vi "Closest Point Delete.vi"(9 "Y in":dbl=359.5 format="%#_13g", 10 "X in":dbl=18.050867335505 format="%#_13g", 11 "All Lines":T1) -> (0 "min index(es)":i32, 1 "Y out":dbl, 2 "X out":dbl, 3 "output array":T1, 5 "Array size":i32)   [LabVIEW 2014]
uses:
  Libraries/Map Data Folder/All-Lines.ctl
  Libraries/Map Data Folder/LineCluster.ctl
  Libraries/Map Data Folder/LineConnection.ctl
  Libraries/Map Data Folder/Map Data.lvlib
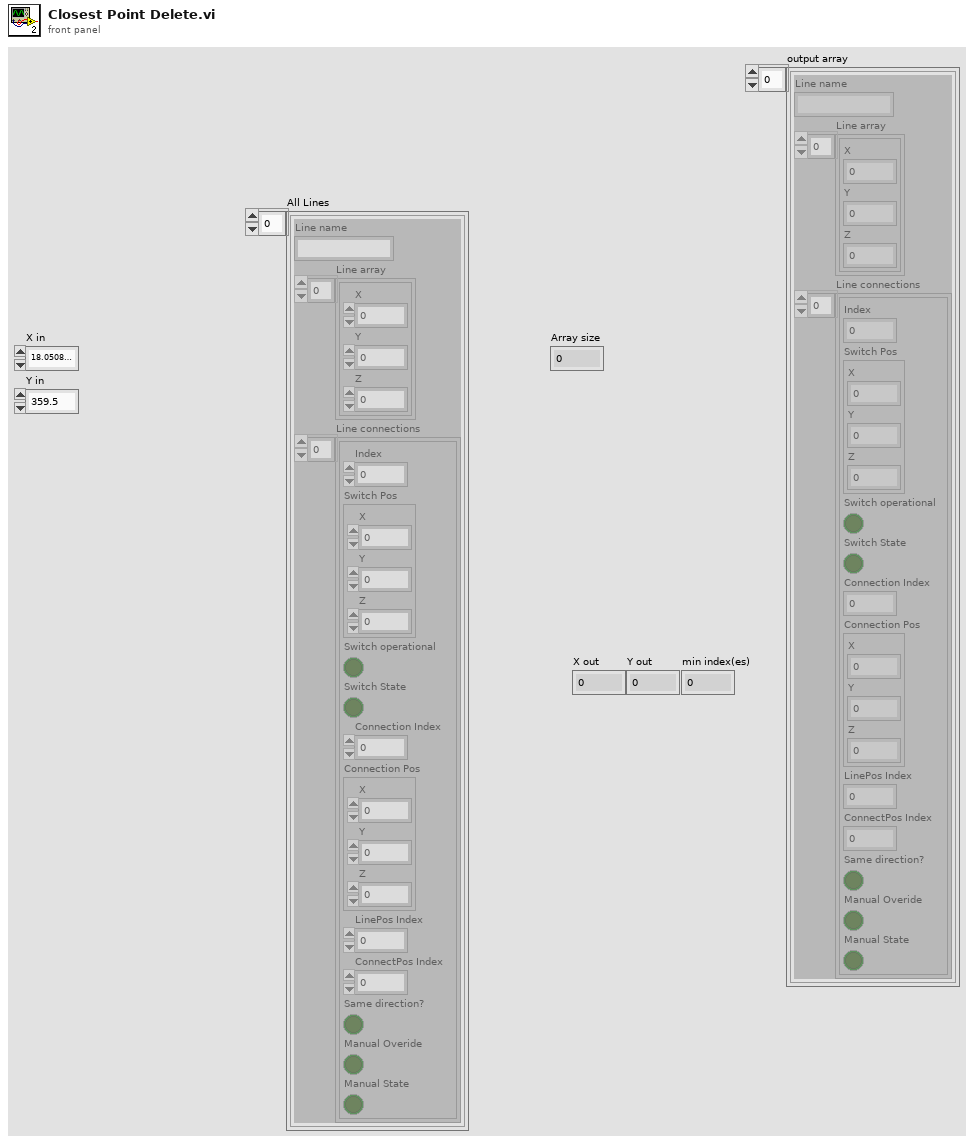
[diagram p1: front panel]
types:
  T1 = typedef "Map Data.lvlib/All-Lines.ctl" = T2[]
  T2 = typedef "Map Data.lvlib/LineCluster.ctl" = cluster{"Line name":string, "Line array":cluster{"X":dbl, "Y":dbl, "Z":dbl}[], "Line connections":T3[]}
  T3 = typedef "Map Data.lvlib/LineConnection.ctl" = cluster{"Index":i32, "Switch Pos":cluster{"X":dbl, "Y":dbl, "Z":dbl}, "Switch operational":bool, "Switch State":bool, "Connection Index":i32, "Connection Pos":cluster{"X":dbl, "Y":dbl, "Z":dbl}, "LinePos Index":i32, "ConnectPos Index":i32, "Same direction?":bool, "Manual Overide":bool, "Manual State":bool}
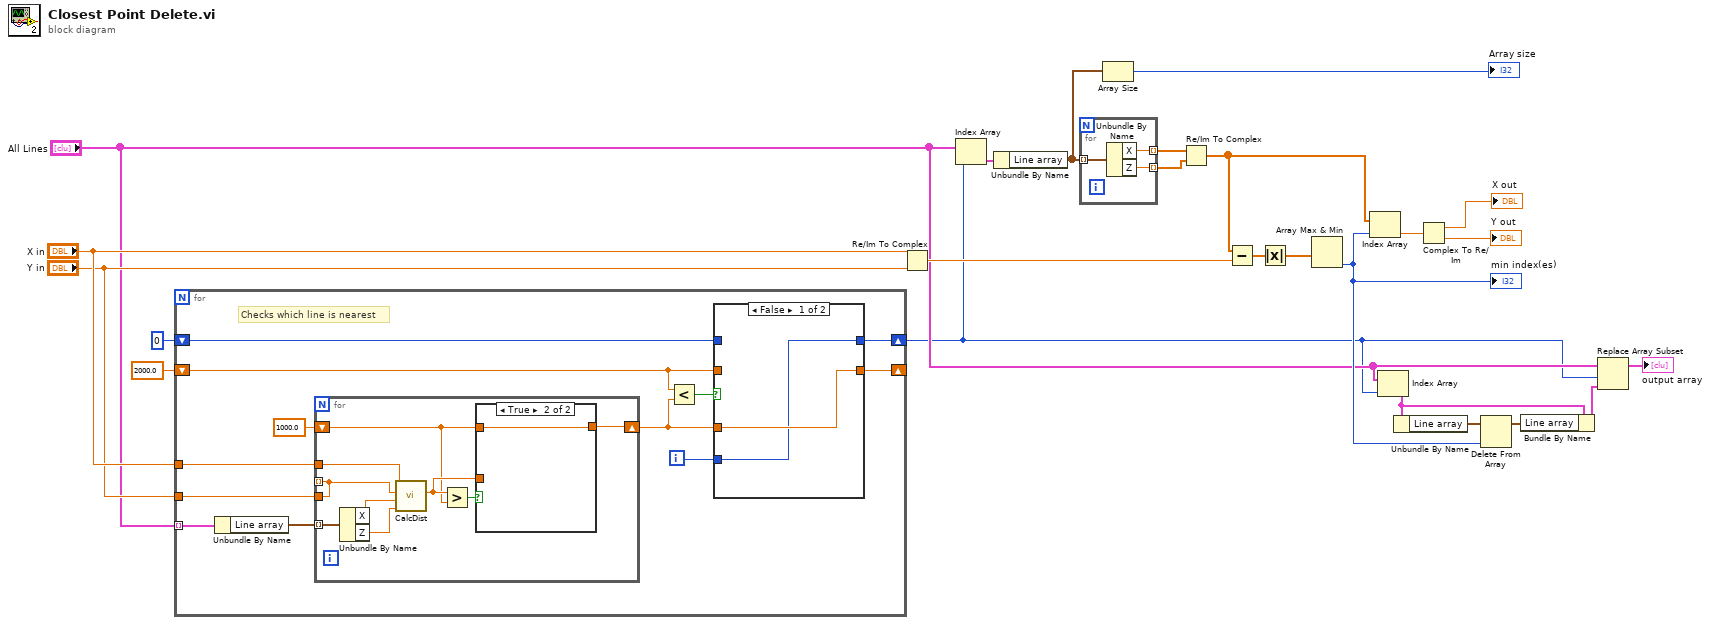
[diagram p0: block diagram]
diagram:
  n1 = for {
    tunnel: "All Lines" -> [w36] mode=indexing
    tunnel: "X in" -> [w34]
    tunnel: "Y in" -> [w33]
    shift-right: [w31] -> _
    shift-left: 2000.0 ("Distance") -> [w27]
    shift-right: [w29] -> w1
    shift-left: 0 -> [w28]
    i -> [w30]
    # "Checks which line is nearest"
    n2 = Unbundle By Name(w36) -> ("Line array"=w35:cluster{"X":dbl, "Y":dbl, "Z":dbl}[])
    n3 = for {
      tunnel: w34 -> [w49]
      tunnel: [w44] -> _ mode=indexing
      tunnel: w35 -> [w48] mode=indexing
      tunnel: w33 -> [w44]
      shift-right: [w41] -> w26
      shift-left: 1000.0 ("Distance") -> [w42]
      n4 = Unbundle By Name(w48) -> ("X"=w45:dbl, "Z"=w46:dbl)
      n5 = call "CalcDist.vi"("Y2"=w46, "X2"=w45, "Y1"=w44, "X1"=w49) -> ("Distance"=w43:dbl)  [unwired: 7 in]
      n6 = Greater?(x=w43, y=w42) -> (0:w47:bool)
      n7 = case shown="True" w47 {
        tunnel: w43 -> [w50 _]
        tunnel: [w50 w51] -> w41
        tunnel: w42 -> [_ w51]
        frame False {
        }
        frame True {
        }
      }
    }
    n8 = Less?(x=w27, y=w26) -> (x < y?=w25:bool)
    n9 = case shown="False" w25 {
      tunnel: w26 -> [w38 _]
      tunnel: [w38 w39] -> w31
      tunnel: w27 -> [_ w39]
      tunnel: w30 -> [w37 _]
      tunnel: [w37 w40] -> w29
      tunnel: w28 -> [_ w40]
      frame False {
      }
      frame True {
      }
    }
  }
  n10 = Re/Im To Complex(1:"Y in", 2:"X in") -> (0:w24:cdb)
  n11 = Index Array(array="All Lines", index=w1) -> (element=w15:T2)
  n12 = Unbundle By Name(w15) -> ("Line array"=w14:cluster{"X":dbl, "Y":dbl, "Z":dbl}[])
  n13 = for {
    tunnel: [w54] -> w18 mode=indexing
    tunnel: [w53] -> w17 mode=indexing
    tunnel: w14 -> [w52] mode=indexing
    n14 = Unbundle By Name(w52) -> ("X"=w54:dbl, "Z"=w53:dbl)
  }
  n15 = Array Size(array=w14) -> (size(s)=→"Array size":i32)
  n16 = Re/Im To Complex(1:w17, 2:w18) -> (0:w16:cdb[])
  n17 = Subtract(x=w16, y=w24) -> (x-y=w20:cdb[])
  n18 = Absolute Value(x=w20) -> (abs(x)=w19:dbl[])
  n19 = Array Max & Min(array=w19) -> (min index (indices)=w12:i32)  [unwired: 3 out]
  "min index(es)" <- w12
  n20 = Index Array(array=w16, index=w12) -> (element=w23:cdb)
  n21 = Index Array(array="All Lines", index=w1) -> (element=w10:T2)
  n22 = Unbundle By Name(w10) -> ("Line array"=w11:cluster{"X":dbl, "Y":dbl, "Z":dbl}[])
  n23 = Complex To Re/Im(x + iy=w23) -> (x=→"X out":dbl, y=→"Y out":dbl)
  n24 = Delete From Array(array=w11, index=w12) -> (array with subset deleted=w9:cluster{"X":dbl, "Y":dbl, "Z":dbl}[])  [unwired: 1 in, 1 out]
  n25 = Bundle By Name(cluster=w10, "Line array"=w9) -> (w8:T2)
  n26 = Replace Array Subset(array="All Lines", new element=w8, index=w1) -> (→"output array":T1)
